vi "Running Avg with Max and Min Excluded.vi"() -> ()   [LabVIEW 2016]
uses:
  Team Code/Robot Global Data.vi
panel:
  out "Difference":dbl
  out "Avg with 2 Mins/Maxs thrown out":dbl
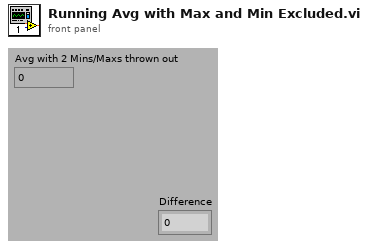
[diagram p1: front panel]
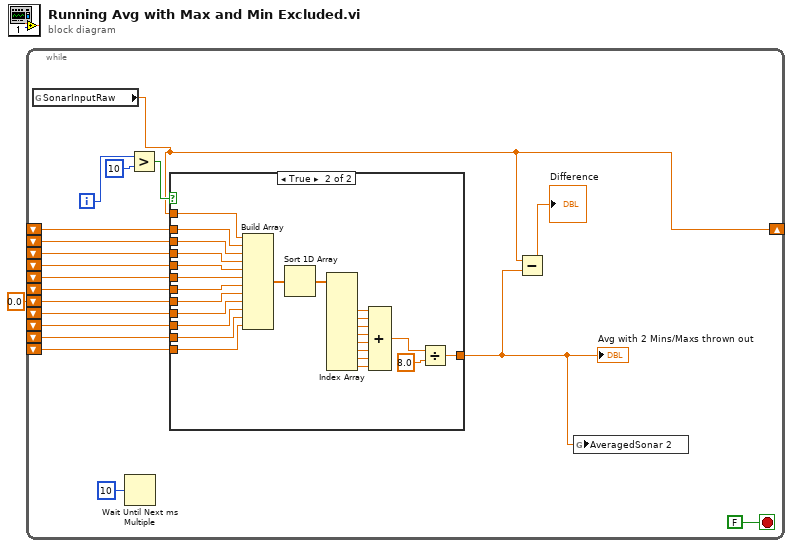
[diagram p0: block diagram]
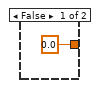
[diagram p2: hidden frame]
diagram:
  w1 = 0.0
  n1 = while {
    shift-right: [w4] -> _
    shift-left: w1 -> [w20]
    shift-left: w1 -> [w19]
    shift-left: w1 -> [w18]
    shift-left: w1 -> [w15]
    shift-left: w1 -> [w14]
    shift-left: w1 -> [w13]
    shift-left: w1 -> [w12]
    shift-left: w1 -> [w11]
    shift-left: w1 -> [w10]
    shift-left: w1 -> [w9]
    shift-left: w1 -> [w8]
    i -> [w7]
    stop <- FALSE stop-if-true
    n2 = global read "Robot Global Data.vi" "SonarInputRaw"() -> (w4:dbl)
    n3 = Wait Until Next ms Multiple(millisecond multiple=u32 10) -> ()  [unwired: 1 out]
    n4 = Greater?(x=w7, y=10) -> (0:w16:bool)
    n5 = case shown="True" w16 {
      tunnel: w20 -> [_ w46]
      tunnel: w19 -> [_ w45]
      tunnel: w18 -> [_ w44]
      tunnel: [0.0 w42] -> w2
      tunnel: w15 -> [_ w41]
      tunnel: w14 -> [_ w40]
      tunnel: w13 -> [_ w39]
      tunnel: w12 -> [_ w38]
      tunnel: w11 -> [_ w37]
      tunnel: w10 -> [_ w36]
      tunnel: w9 -> [_ w35]
      tunnel: w8 -> [_ w34]
      tunnel: w4 -> [_ w22]
      frame False {
      }
      frame True {
        n6 = Build Array(w22, w46, w45, w44, w41, w40, w39, w38, w37, w36, w35, w34) -> (w33:dbl[])
        n7 = Sort 1D Array(array=w33) -> (sorted array=w32:dbl[])
        n8 = Index Array(array=w32) -> (element #3=w23:dbl, element #4=w31:dbl, element #5=w30:dbl, element #6=w29:dbl, element #7=w28:dbl, element #8=w27:dbl, element #9=w26:dbl, element #10=w25:dbl)  [unwired: 10 in, 2 out]
        n9 = Compound Arithmetic op=ADD(w23, w31, w30, w29, w28, w27, w26, w25) -> (w24:dbl)
        n10 = Divide(x=w24, y=8.0) -> (x/y=w42:dbl)
      }
    }
    "Avg with 2 Mins/Maxs thrown out" <- w2
    n11 = Subtract(x=w4, y=w2) -> (x-y=→"Difference":dbl)
    n12 = global write "Robot Global Data.vi" "AveragedSonar 2"(w2) -> ()
  }
